vi "oa_Check Spectrum Settings [OPS] (1 Channel).vi"(6 "spectrum settings":cluster{"window type":u32, "block size":i32}={"window type"=1, "block size"=400} {"block size" min=2; "window type" items=["None"=0, "Hanning"=1, "Hamming"=2, "Blackman-Harris"=3, "Exact Blackman"=4, "Blackman"=5, "Flat Top"=6, "4 Term B-Harris"=7, "7 Term B-Harris"=8, "Low Sidelobe"=9, "Gaussian"=62]}, 8 "error in (no error)":errorcluster, 11 "resampled signal":cluster{"r0":dbl, "dr":dbl, "Y":dbl[]} {"r0" format="%.2p"; "dr" format="%.2p"; "Y" format="%.2f"}) -> (0 "error out":errorcluster, 2 "parameter changed":bool, 3 "resampled signal dup":cluster{"r0":dbl, "dr":dbl, "Y":dbl[]} {"r0" format="%.2p"; "dr" format="%.2p"; "Y" format="%.2f"})   [LabVIEW 2017, in "SoundVib_Resampling.lvlib"]
uses:
  <vilib>/addons/Sound and Vibration/Order Analysis/Resample Order Tracking/SoundVib_Resampling.lvlib
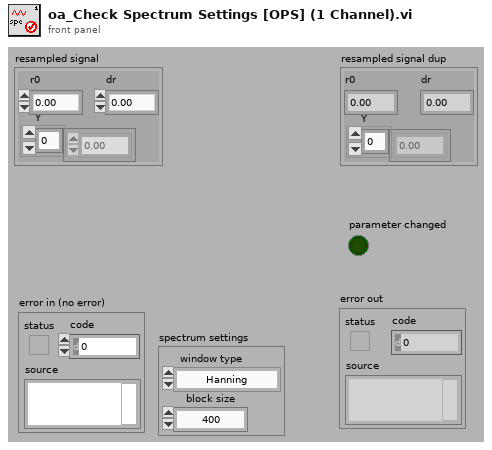
[diagram p1: front panel]
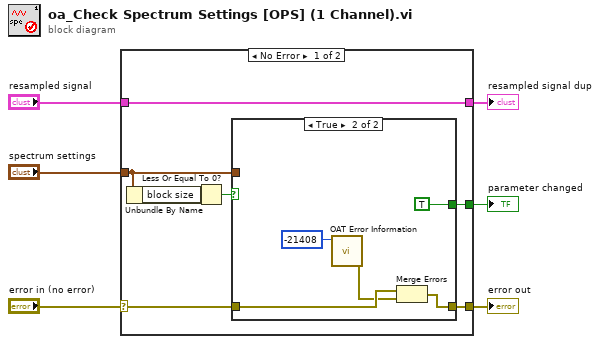
[diagram p0: block diagram]
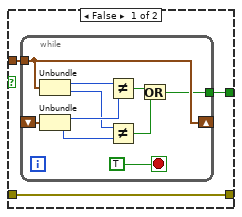
[diagram p2: hidden frame]
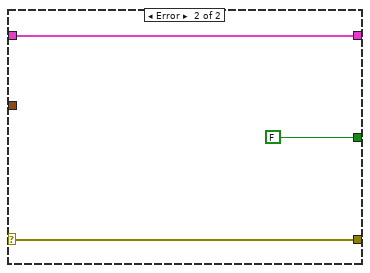
[diagram p3: hidden frame]
diagram:
  n1 = case shown="No Error" "error in (no error)" {
    selector: "error in (no error)" -> [w8 w34]
    tunnel: [w7 w34] -> w5
    tunnel: "resampled signal" -> [w13 w33]
    tunnel: [w13 w33] -> w3
    tunnel: "spectrum settings" -> [w11 _]
    tunnel: [w12 FALSE] -> w1
    frame No Error {
      n2 = Unbundle By Name(w11) -> ("block size"=w10:i32)
      n3 = Less Or Equal To 0?(x=w10) -> (x <= 0?=w9:bool)
      n4 = case shown="True" w9 {
        tunnel: [w16 TRUE] -> w12
        tunnel: w11 -> [w15 _]
        tunnel: w8 -> [w14 w29]
        tunnel: [w14 w27] -> w7
        frame False {
          n5 = while {
            tunnel: w15 -> [w25]
            shift-right: [w25] -> _
            shift-left: _ -> [w23]
            tunnel: [w17] -> w16
            stop <- TRUE stop-if-true
            n6 = Unbundle(w25) -> ("window type"=w24:u32, "block size"=w21:i32)
            n7 = Unbundle(w23) -> ("window type"=w22:u32, "block size"=w20:i32)
            n8 = Not Equal?(x=w24, y=w22) -> (x != y?=w19:bool)
            n9 = Not Equal?(x=w21, y=w20) -> (x != y?=w18:bool)
            n10 = Or(x=w19, y=w18) -> (x .or. y?=w17:bool)
          }
        }
        frame True {
          n11 = call <vilib>:"OAT Error Information.vi"("error code"=-21408) -> ("error out"=w28:errorcluster)  [unwired: 6 in]
          n12 = Merge Errors(w29, w28) -> (w27:errorcluster)
        }
      }
    }
    frame Error {
    }
  }
  "resampled signal dup" <- w3
  "error out" <- w5
  "parameter changed" <- w1
